vi "peak detector.vi"(11 "Filtered Signal":dynamicdata(waveform)) -> (1 "Locations":dbl[](array[numeric]), 2 "Waveform":waveform(dbl), 3 "Y":dbl[](array[numeric]))   [LabVIEW 2021]
uses:
  <vilib>/Waveform/WDTOps.llb/WDT Get XY Value DBL.vi
  <vilib>/Analysis/NI_AAL_SigProc.lvlib
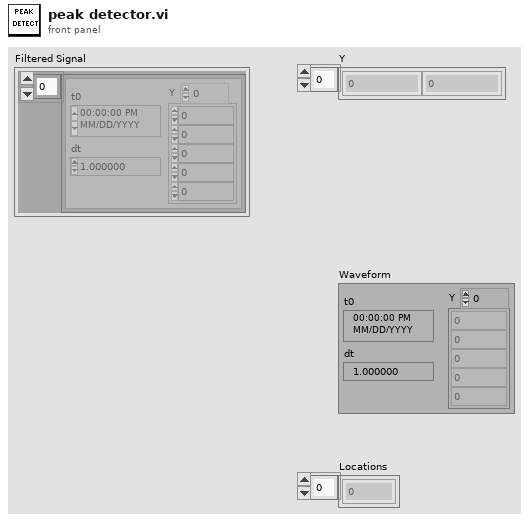
[diagram p1: front panel]
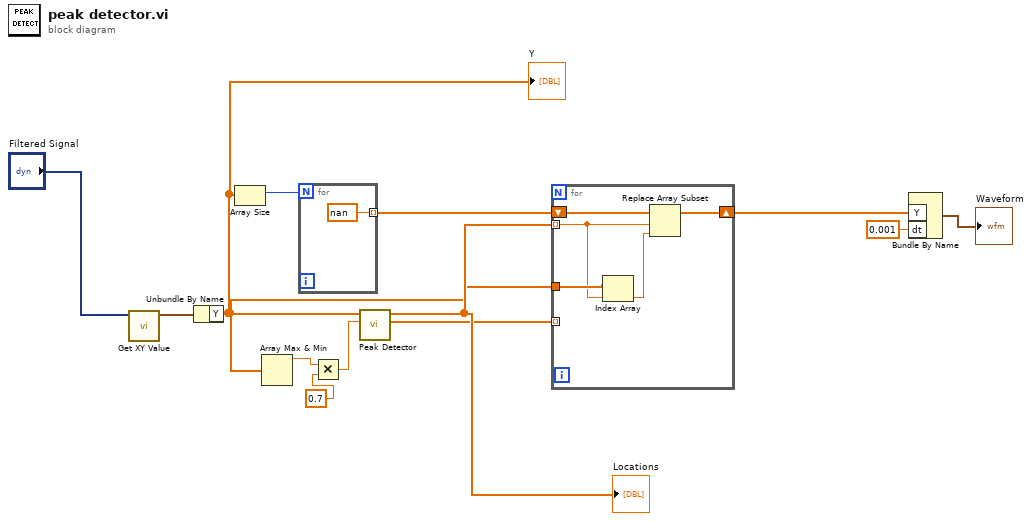
[diagram p0: block diagram]
diagram:
  n1 = call-poly <vilib>:"Get XY Value.vi"("waveform in"="Filtered Signal") -> ("waveform out"=w3:waveform(dbl))  [unwired: 6 in, 4 out]
  n2 = Unbundle By Name(w3) -> ("Y"=w1:dbl[])
  "Y" <- w1
  n3 = Array Size(array=w1) -> (size(s)=w5:i32)
  n4 = Array Max & Min(array=w1) -> (max value=w7:dbl)  [unwired: 3 out]
  n5 = for {
    N: w5 -> [_]
    tunnel: [nan] -> w4 mode=indexing
  }
  n6 = Multiply(x=w7, y=0.7) -> (x*y=w2:dbl)
  n7 = call <vilib>:"Peak Detector.vi"("threshold"=w2, "X"=w1) -> ("Amplitudes"=w9:dbl[], "Locations"=w10:dbl[])  [unwired: 5 in, 3 out]
  "Locations" <- w10
  n8 = for {
    tunnel: w10 -> [w16] mode=indexing
    shift-right: [w18] -> w6
    shift-left: w4 -> [w19]
    tunnel: w9 -> [_] mode=indexing
    tunnel: w1 -> [w17]
    n9 = Index Array(array=w17, index=w16) -> (element=w15:dbl)
    n10 = Replace Array Subset(array=w19, new element=w15, index=w16) -> (w18:dbl[])
  }
  n11 = Bundle By Name("Y"=w6, "dt"=0.001) -> (→"Waveform":waveform(dbl))  [unwired: 1 in]
